vi "Test Insert Image ARGB.vi"(8 "error in (no error)":errorcluster, 11 "Test Case In":refnum<class "01_Image.lvclass">) -> (0 "error out":errorcluster, 3 "Test Case Out":refnum<class "01_Image.lvclass">)   [LabVIEW 2020, in "test.lvlib" / "01_Image.lvclass"]
uses:
  01_Image.lvclass
  C:/Program Files (x86)/National Instruments/LabVIEW 2026/vi.lib/Astemes/LUnit/Test Case.lvclass
  common/Image Size (Integer).ctl
  image/ARGB Colour.ctl
  <vilib>/Astemes/LUnit/Test Case.lvclass/Test Case.ctl
  image/New Image (ARGB Preallocated).vi
  image/Draw Image to Picture (ARGB).vi
  4993e8ee-a06a-463a-9684-69129f64d5ce.vi
  image/Copy Array to Image.vi
  image/Copy Array to Image (ARGB).vi
  image/New Image (ARGB Preallocated).vi/3321fa97-f432-4e1e-8db9-a0df79aed21b.vi
  image/ARGB Colour to U32 Pixel Value.vi
  image/Insert Image (ARGB).vi/5e3288c8-ee88-4cfe-89cf-31ceca475f5a.vi
  image/Draw Image to Picture (ARGB).vi/8cd07b1b-062e-4fe4-9e87-2eb3dc89fe0e.vi
  <vilib>/Astemes/LUnit/Core/LUnit Test Case/Private/Append Pass Result.vi
  <vilib>/Astemes/LUnit/Core/LUnit Test Case/Private/Append Fail Result.vi
  4993e8ee-a06a-463a-9684-69129f64d5ce.vi/9c5d11cd-9439-4240-a1ee-d9baace9c924.vi
  <vilib>/Astemes/LUnit/Core/LUnit Test Case/Private/Run In UI.vi
  <vilib>/Utility/error.llb/Clear Errors.vi
  <vilib>/Utility/error.llb/Error Cluster From Error Code.vi
  <vilib>/picture/pixmap.llb/Flatten Pixmap.vi
  image/image.lvlib
  common/common.lvlib
panel:
  out "Picture":picture
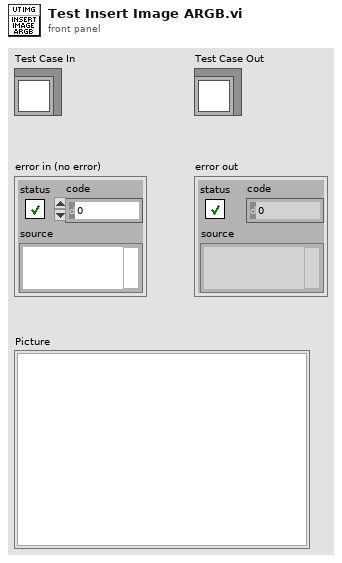
[diagram p1: front panel]
types:
  T1 = typedef "image.lvlib/ARGB Colour.ctl" = cluster{"Alpha":u8, "RGB":u32}
  T2 = typedef "common.lvlib/Image Size (Integer).ctl" = cluster{"Width":u16, "Height":u16}
  T3 = typedef "image.lvlib/ARGB Image.ctl" = refnum<data-value>
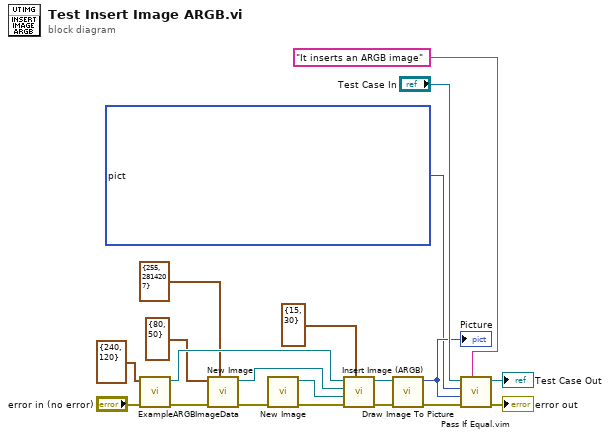
[diagram p0: block diagram]
diagram:
  n1 = call "ExampleARGBImageData.vi"("error in (no error)"="error in (no error)", "Image Size"=T2 {"Width"=240, "Height"=120} ("Preallocated Image Size (Default - 0,0)")) -> ("error out"=w8:errorcluster, "Data Value Reference out"=w14:T3)  [unwired: 6 in, 2 out]
  n2 = call-poly "New Image.vi"("Colour (Default: Black)"=T1 {"Alpha"=255, "RGB"=2814207}, "error in (no error)"=w8, "Preallocated Image Size (Default: 0,0)"=T2 {"Width"=80, "Height"=50} ("Preallocated Image Size")) -> ("error out"=w7:errorcluster, "ARGB Image"=w6:T3)  [unwired: 7 in]
  n3 = call-poly "New Image.vi"("error in (no error)"=w7) -> ("error out"=w16:errorcluster, "ARGB Image"=w11:T3)  [unwired: 9 in]
  n4 = call "Insert Image (ARGB).vi"("Offset (Default: 0,0)"=T2 {"Width"=15, "Height"=30}, "error in (no error)"=w16, "ARGB Image Destination in"=w11, "ARGB Image Child in"=w6, "ARGB Image Parent in"=w14) -> ("error out"=w4:errorcluster, "ARGB Image Destination"=w10:T3)  [unwired: 5 in]
  n5 = call-poly "Draw Image To Picture.vi"("error in (no error)"=w4, "ARGB Image Source in"=w10) -> ("error out"=w3:errorcluster, "Picture"=w2:picture)  [unwired: 8 in]
  "Picture" <- w2
  n6 = call "Pass If Equal.vim"("Description"="It inserts an ARGB image", "error in (no error)"=w3, "Actual"=w2, "Expected"=picture bytes[86430] ("Picture"), "LUnit Test Case In"="Test Case In") -> ("error out"=→"error out":errorcluster, "LUnit Test Case Out"=→"Test Case Out":refnum<class "01_Image.lvclass">)  [unwired: 5 in]
